vi "Begin.vi"() -> (0 "error out":errorcluster, 1 "CameraDevRef":T1)   [LabVIEW 2011]
doc: "Called before other user functions, this VI is expected to open initial I/O refnums, load in file data, and do all program initialization. Notice that the <B>error out</B> terminal is simply used for data flow. Wiring it to other structures or subVIs ensures that this VI runs first."
uses:
  <vilib>/Rock Robotics/WPI/Camera/WPI_CameraDevRef.ctl
  <vilib>/Rock Robotics/SystemInterfaces/DIO/FPGA_DIOPWMChannel.ctl
  <vilib>/Rock Robotics/WPI/Joystick/WPI_JoystickDeviceEnum.ctl
  <vilib>/Rock Robotics/WPI/Relay/WPI_RelayDirection.ctl
  <vilib>/Rock Robotics/SystemInterfaces/DIO/FPGA_DIORelayChannel.ctl
  <vilib>/Rock Robotics/SystemInterfaces/Typedef/FPGA_TypedefDigitalModule.ctl
  <vilib>/Rock Robotics/SystemInterfaces/AI/FPGA_AIChannel.ctl
  <vilib>/Rock Robotics/WPI/MotorControl/WPI_MotorControlOpen Jaguar.vi
  <vilib>/Rock Robotics/WPI/MotorControl/WPI_MotorControlOpen Victor.vi
  Robot Global Data.vi
panel:
  out "Global: Auton Files":string[](array[string])
  out "Global: Auton Array":dbl[][](array[numeric])
  out "Global: Current Auton File":string
  out "Global: Number of Auton Files":i64
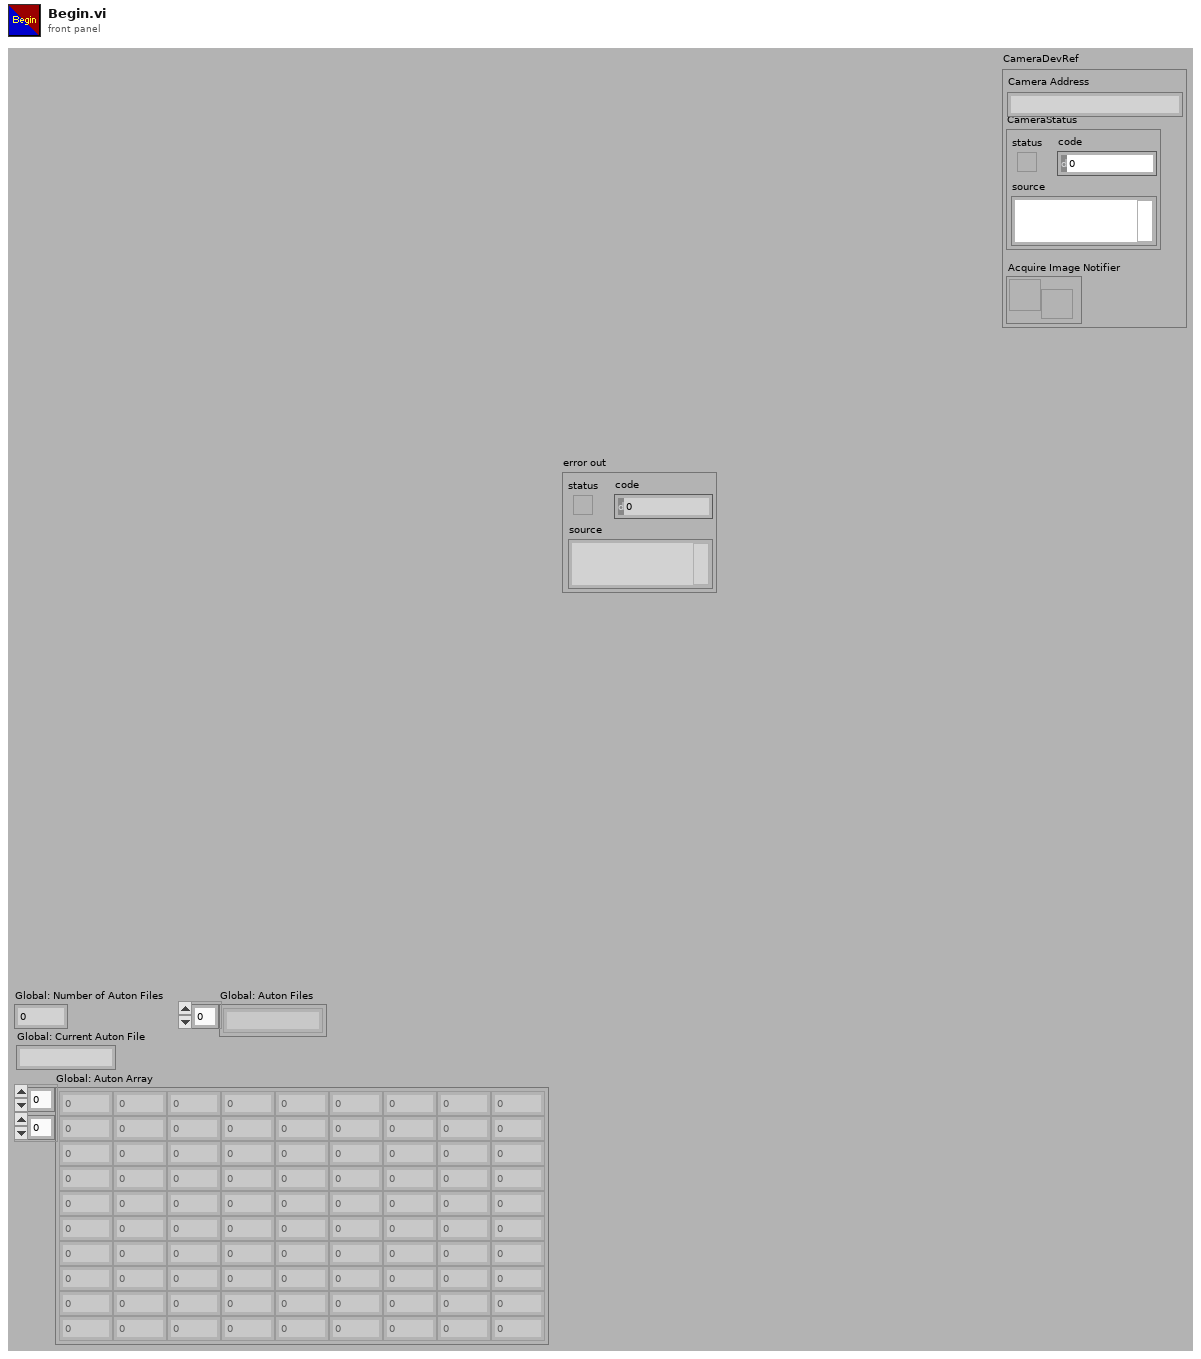
[diagram p1: front panel]
types:
  T1 = typedef "WPI_CameraDevRef.ctl" = cluster{"Camera Address":string, "CameraStatus":errorcluster, "Acquire Image Notifier":refnum<notifier>}
  T2 = typedef "FPGA_AIChannel.ctl" = enum8{"AI 1", "AI 2", "AI 3", "AI 4", "AI 5", "AI 6", "AI 7", "AI 8", "Invalid"}
  T3 = typedef "FPGA_TypedefDigitalModule.ctl" = enum16{"Digital Module 1", "Digital Module 2"}
  T4 = typedef "FPGA_DIORelayChannel.ctl" = enum8{"Relay 1", "Relay 2", "Relay 3", "Relay 4", "Relay 5", "Relay 6", "Relay 7", "Relay 8", "Invalid"}
  T5 = typedef "WPI_RelayDirection.ctl" = enum16{"Both directions", "Forward only", "Reverse only"}
  T6 = typedef "WPI_JoystickDeviceEnum.ctl" = enum16{"USB 1", "USB 2", "USB 3", "USB 4", "Kinect 1", "Kinect 2"}
  T7 = typedef "FPGA_DIOPWMChannel.ctl" = enum8{"PWM 1", "PWM 2", "PWM 3", "PWM 4", "PWM 5", "PWM 6", "PWM 7", "PWM 8", "PWM 9", "PWM 10", "Invalid"}
  T8 = typedef "WPI_CameraImageSize.ctl" = enum16{"640x480", "320x240", "160x120"}
  T9 = cluster{"fps":i32, "compression":i32, "Image Size":T8}
  T10 = typedef "WPI_CameraWhite Balance Values.ctl" = enum16{"Auto", "Fixed indoor", "Fixed outdoor 1", "Fixed outdoor 2", "Fixed fluorescent 1", "Fixed fluorescent 2", "Hold current"}
  T11 = typedef "WPI_ServoDeviceRef.ctl" = cluster{"DeviceStatus":errorcluster, "Digital Module":T3, "PWM Channel":T7, "DeadBand":T12}
  T12 = typedef "WPI_PWMDeadband.ctl" = cluster{"Name":string, "maxPositivePwm":i32, "minPositivePwm":i32, "centerPwm":i32, "maxNegativePwm":i32, "minNegativePwm":i32, "angularRange":u16}
  T13 = typedef "WPI_MotorControlDeviceRef.ctl" = cluster{"DeviceStatus":errorcluster, "Type":enum16{"PWM", "CAN"}, "PWM":cluster{"Digital Module":T3, "PWM Channel":T7, "DeadBand":T12}, "CAN":cluster{"Device Number":u8, "Control Mode":T14, "Semaphore":T15, "Max Vout":dbl}, "Invert":bool, "TransformRef":T16, "InvTransformRef":T16}
  T14 = typedef "WPI_CANJaguar_ControlMode.ctl" = enum8{"Percent VBus", "Current", "Speed", "Position", "Voltage"}
  T15 = typedef "Semaphore RefNum" = refnum<k1>
  T16 = typedef "WPI_PWMTransform_ConPane.ctl" = refnum<vi>
  T17 = typedef "WPI_CameraExposure Values.ctl" = enum16{"Auto", "Flicker-free 50 Hz", "Flicker-free 60 Hz", "Hold current"}
  T18 = typedef "WPI_AnalogChannelDevRef.ctl" = cluster{"DevStatus":errorcluster, "Analog Module":T19, "Analog Channel":T2}
  T19 = typedef "FPGA_TypedefAnalogModule.ctl" = enum16{"Analog Module 1", "Analog Module 2"}
  T20 = typedef "WPI_JoystickDevRef.ctl" = cluster{"Device":T6}
  T21 = typedef "WPI_RelayDevRef.ctl" = cluster{"DevStatus":errorcluster, "Relay Channel":T4, "Digital Module":T3, "Relay Direction":T5}
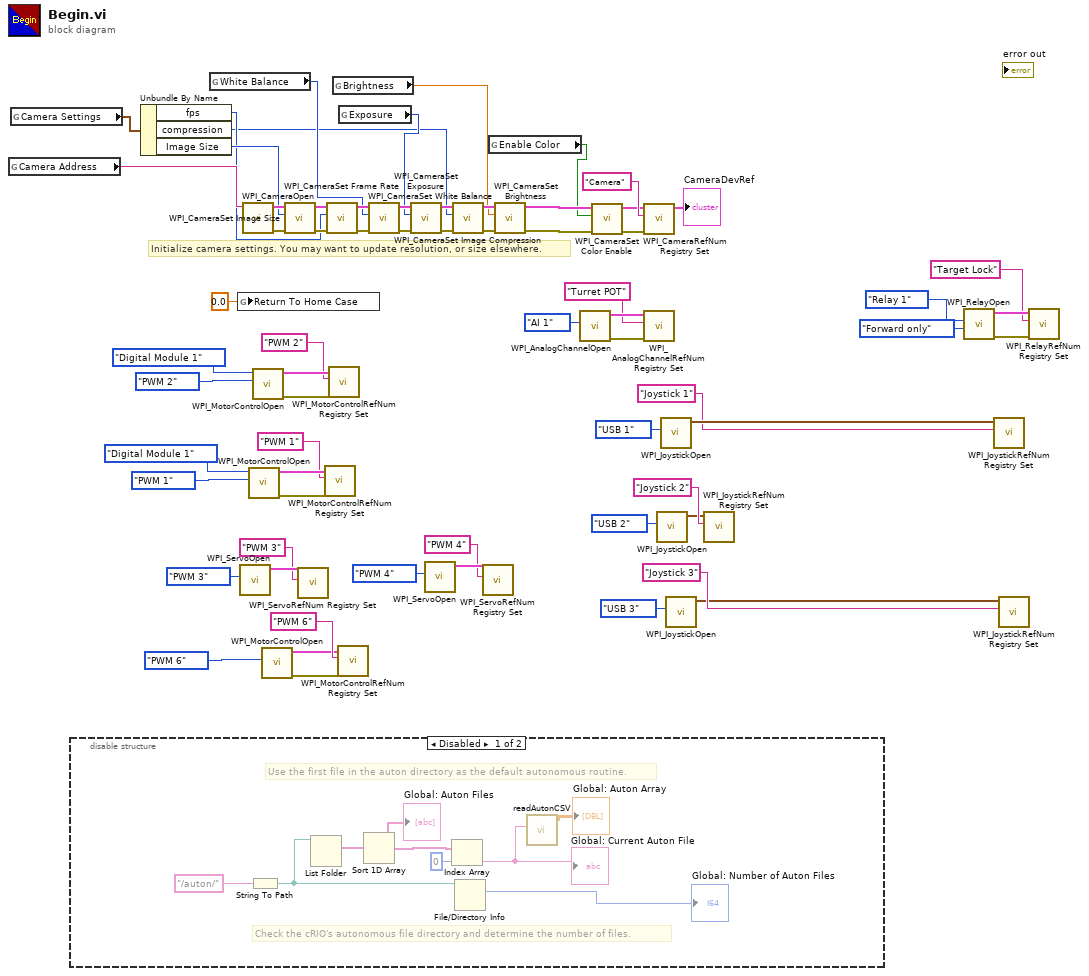
[diagram p0: block diagram]
diagram:
  # "Initialize camera settings. You may want to update resolution, or size elsewhere."
  n1 = global read "Robot Global Data.vi" "Camera Address"() -> (w53:string)
  n2 = global read "Robot Global Data.vi" "Camera Settings"() -> (w25:T9)
  n3 = disable-structure shown="Disabled" {
    frame Disabled {
      # "Check the cRIO's autonomous file directory and determine the number of files."
      # "Use the first file in the auton directory as the default autonomous routine."
      n4 = String To Path(string="/auton/") -> (path=w73:path)
      n5 = List Folder(path=w73) -> (filenames=w72:string[])  [unwired: 1 in, 5 out]
      n6 = Sort 1D Array(array=w72) -> (sorted array=w70:string[])
      "Global: Auton Files" <- w70
      n7 = Index Array(array=w70, index=0) -> (element=w68:string)
      "Global: Current Auton File" <- w68
      n8 = File/Directory Info(path=w73) -> (size=→"Global: Number of Auton Files":i64)  [unwired: 1 in, 6 out]
      n9 = call "readAutonCSV.vi"("AutonFile"=w68) -> ("AutonArray"=→"Global: Auton Array":dbl[][])  [unwired: 7 in]
    }
    frame Enabled {
    }
  }
  n10 = Unbundle By Name(w25) -> ("fps"=w23:i32, "compression"=w20:i32, "Image Size"=w24:T8)
  n11 = global read "Robot Global Data.vi" "White Balance"() -> (w22:T10)
  n12 = global write "Robot Global Data.vi" "Return To Home Case"(0.0 ("Return To Home Case")) -> ()
  n13 = call <vilib>:"WPI_ServoOpen.vi"("PWM Channel"=FPGA_DIOPWMChannel."PWM 3") -> ("ServoDeviceRef"=w39:T11)  [unwired: 9 in, 1 out]
  n14 = call <vilib>:"WPI_CameraOpen.vi"("Camera Address"=w53) -> ("error out"=w59:errorcluster, "CameraDevRef"=w60:T1)  [unwired: 1 in, 8 out]
  n15 = call-poly <vilib>:"WPI_MotorControlOpen.vi"("PWM Channel"=FPGA_DIOPWMChannel."PWM 1", "Digital Module (Module 1)"=FPGA_TypedefDigitalModule."Digital Module 1") -> ("error out"=w45:errorcluster, "MotorControlDeviceRef"=w48:T13)  [unwired: 8 in]
  n16 = call-poly <vilib>:"WPI_MotorControlOpen.vi"("PWM Channel"=FPGA_DIOPWMChannel."PWM 2", "Digital Module (Module 1)"=FPGA_TypedefDigitalModule."Digital Module 1") -> ("error out"=w46:errorcluster, "MotorControlDeviceRef"=w51:T13)  [unwired: 8 in]
  n17 = call-poly <vilib>:"WPI_MotorControlOpen.vi"("PWM Channel"=FPGA_DIOPWMChannel."PWM 6") -> ("error out"=w34:errorcluster, "MotorControlDeviceRef"=w32:T13)  [unwired: 9 in]
  n18 = call <vilib>:"WPI_CameraSet Image Size.vi"("error in (no error)"=w59, "Image Size"=w24, "CameraDevRef"=w60) -> ("error out"=w58:errorcluster, "CameraDevRef Out"=w61:T1)  [unwired: 7 out]
  n19 = call <vilib>:"WPI_ServoRefNum Registry Set.vi"("refnum name"="PWM 3", "ServoDeviceRef"=w39) -> ()  [unwired: 8 in, 2 out]
  n20 = call <vilib>:"WPI_MotorControlRefNum Registry Set.vi"("error in (no error)"=w45, "refnum name"="PWM 1", "MotorControlDevRef"=w48) -> ()  [unwired: 7 in, 2 out]
  n21 = call <vilib>:"WPI_CameraSet Frame Rate.vi"("error in (no error)"=w58, "Frame Rate (fps)"=w23, "CameraDevRef"=w61) -> ("error out"=w57:errorcluster, "CameraDevRef Out"=w63:T1)  [unwired: 7 out]
  n22 = call <vilib>:"WPI_MotorControlRefNum Registry Set.vi"("error in (no error)"=w46, "refnum name"="PWM 2", "MotorControlDevRef"=w51) -> ()  [unwired: 7 in, 2 out]
  n23 = global read "Robot Global Data.vi" "Brightness"() -> (w19:dbl)
  n24 = call <vilib>:"WPI_MotorControlRefNum Registry Set.vi"("error in (no error)"=w34, "refnum name"="PWM 6", "MotorControlDevRef"=w32) -> ()  [unwired: 7 in, 2 out]
  n25 = global read "Robot Global Data.vi" "Exposure"() -> (w21:T17)
  n26 = call <vilib>:"WPI_CameraSet White Balance.vi"("error in (no error)"=w57, "White Balance"=w22, "CameraDevRef"=w63) -> ("error out"=w56:errorcluster, "CameraDevRef Out"=w62:T1)  [unwired: 7 out]
  n27 = call <vilib>:"WPI_CameraSet Exposure.vi"("error in (no error)"=w56, "Exposure"=w21, "CameraDevRef"=w62) -> ("error out"=w55:errorcluster, "CameraDevRef Out"=w65:T1)  [unwired: 7 out]
  n28 = call <vilib>:"WPI_ServoOpen.vi"("PWM Channel"=FPGA_DIOPWMChannel."PWM 4") -> ("ServoDeviceRef"=w37:T11)  [unwired: 9 in, 1 out]
  n29 = call <vilib>:"WPI_CameraSet Image Compression.vi"("error in (no error)"=w55, "Compression"=w20, "CameraDevRef"=w65) -> ("error out"=w54:errorcluster, "CameraDevRef Out"=w64:T1)  [unwired: 7 out]
  n30 = call <vilib>:"WPI_ServoRefNum Registry Set.vi"("refnum name"="PWM 4", "ServoDeviceRef"=w37) -> ()  [unwired: 8 in, 2 out]
  n31 = global read "Robot Global Data.vi" "Enable Color"() -> (w14:bool)
  n32 = call <vilib>:"WPI_CameraSet Brightness.vi"("error in (no error)"=w54, "Brightness"=w19, "CameraDevRef"=w64) -> ("error out"=w17:errorcluster, "CameraDevRef Out"=w18:T1)  [unwired: 7 out]
  n33 = call <vilib>:"WPI_AnalogChannelOpen.vi"("Analog Channel"=FPGA_AIChannel."AI 1") -> ("error out"=w4:errorcluster, "AIDeviceRef"=w5:T18)  [unwired: 9 in]
  n34 = call <vilib>:"WPI_CameraSet Color Enable.vi"("error in (no error)"=w17, "Color Enabled"=w14, "CameraDevRef"=w18) -> ("error out"=w15:errorcluster, "CameraDevRef Out"=w16:T1)  [unwired: 7 in]
  n35 = call <vilib>:"WPI_CameraRefNum Registry Set.vi"("error in (no error)"=w15, "refnum name"="Camera", "CameraDevRef"=w16) -> ("CameraDevRef"=→"CameraDevRef":T1)  [unwired: 8 out]
  n36 = call <vilib>:"WPI_AnalogChannelRefNum Registry Set.vi"("error in (no error)"=w4, "refnum name"="Turret POT", "AIDeviceRef"=w5) -> ()  [unwired: 7 in, 2 out]
  n37 = call <vilib>:"WPI_JoystickOpen.vi"("JoystickDevice"=WPI_JoystickDeviceEnum."USB 2") -> ("JoystickDevRef"=w41:T20)  [unwired: 10 in]
  n38 = call <vilib>:"WPI_JoystickOpen.vi"("JoystickDevice"=WPI_JoystickDeviceEnum."USB 1") -> ("JoystickDevRef"=w44:T20)  [unwired: 10 in]
  n39 = call <vilib>:"WPI_JoystickOpen.vi"("JoystickDevice"=WPI_JoystickDeviceEnum."USB 3") -> ("JoystickDevRef"=w29:T20)  [unwired: 10 in]
  n40 = call <vilib>:"WPI_JoystickRefNum Registry Set.vi"("refnum name"="Joystick 2", "JoystickDevRef"=w41) -> ()  [unwired: 8 in, 2 out]
  n41 = call <vilib>:"WPI_RelayOpen.vi"("Relay Direction"=WPI_RelayDirection."Forward only", "Relay Channel"=FPGA_DIORelayChannel."Relay 1") -> ("error out"=w11:errorcluster, "RelayDevRef"=w12:T21)  [unwired: 8 in]
  n42 = call <vilib>:"WPI_JoystickRefNum Registry Set.vi"("refnum name"="Joystick 1", "JoystickDevRef"=w44) -> ()  [unwired: 8 in, 2 out]
  n43 = call <vilib>:"WPI_JoystickRefNum Registry Set.vi"("refnum name"="Joystick 3", "JoystickDevRef"=w29) -> ()  [unwired: 8 in, 2 out]
  n44 = call <vilib>:"WPI_RelayRefNum Registry Set.vi"("error in (no error)"=w11, "refnum name"="Target Lock", "RelayDevRef"=w12) -> ()  [unwired: 7 in, 2 out]
